vi "Begin.vi"(8 "error in":errorcluster) -> (0 "error out":errorcluster)   [LabVIEW 2017]
doc: "Called before other user functions, this VI is expected to open initial I/O refnums, load in file data, and do all program initialization. Notice that the <B>error out</B> terminal is simply used for data flow. Wiring it to other structures or subVIs ensures that this VI runs first."
uses:
  <vilib>/Rock Robotics/WPI/DriverStation/WPI_DriverStationRobotMode2.ctl
  <vilib>/Rock Robotics/WPI/Joystick/WPI_JoystickDeviceEnum.ctl
  <vilib>/Rock Robotics/WPI/ThirdParty/Phoenix-LabVIEW/Motor Controller/Controls/CTRE_Phoenix_MotorControl_NeutralMode.ctl
  <vilib>/Rock Robotics/WPI/ThirdParty/Phoenix-LabVIEW/Motor Controller/Controls/CTRE_Phoenix_MotorControl_FeedbackDevice.ctl
  Robot Global Data.vi
  <vilib>/Rock Robotics/WPI/ThirdParty/Phoenix-LabVIEW/Pigeon IMU/CTRE_PigeonIMU_Open_TalonSRX.vi
panel:
  in  "Invert? 2":bool=TRUE
  in  "Invert?":bool
  in  "PhaseSensor 2":bool
  in  "PhaseSensor":bool=TRUE
  in  "6 motors?":bool
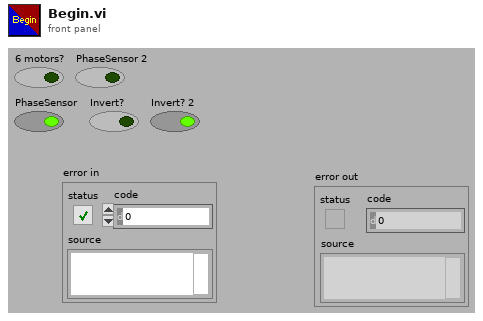
[diagram p1: front panel]
types:
  T1 = typedef "CTRE_Phoenix_MotorControl_FeedbackDevice.ctl" = i8
  T2 = typedef "CTRE_Phoenix_MotorControl_NeutralMode.ctl" = enum8{"EEPROMSetting", "Override to Coast", "Override to Brake"}
  T3 = typedef "WPI_JoystickDeviceEnum.ctl" = enum16{"USB 0", "USB 1", "USB 2", "USB 3", "USB 4", "USB 5"}
  T4 = typedef "WPI_DriverStationRobotMode2.ctl" = enum16{"Autonomous Disabled", "Autonomous Enabled", "Teleop Disabled", "Teleop Enabled", "Disconnected", "Finish", "Test Disabled", "Test Enabled", "Emergency Stopped"}
  T5 = typedef "WPI_MotorControlDeviceRef.ctl" = cluster{"DeviceStatus":errorcluster, "Type":T6, "PWM":cluster{"PWM Channel":T7, "DeadBand":T8}, "CAN":cluster{"Device Number":u8, "SetOutput VI Ref":variant, "GetOutput VI Ref":variant, "Enable VI Ref":variant, "Disable VI Ref":variant, "Data":variant}, "Invert":bool, "DIO PWM":cluster{"PWM \"Enable\" Channel":T7, "DIOChannel":T9, "PWM Rate":dbl}}
  T6 = typedef "WPI_MotorControlType.ctl" = enum16{"PWM", "CAN", "DIO PWM"}
  T7 = typedef "FPGA_DIOPWMChannel.ctl" = enum8{"PWM 0", "PWM 1", "PWM 2", "PWM 3", "PWM 4", "PWM 5", "PWM 6", "PWM 7", "PWM 8", "PWM 9", "PWM MXP 0", "PWM MXP 1", "PWM MXP 2", "PWM MXP 3", "PWM MXP 4", "PWM MXP 5", "PWM MXP 6", "PWM MXP 7", "PWM MXP 8", "PWM MXP 9", "Invalid"}
  T8 = typedef "WPI_PWMDeadband.ctl" = cluster{"Name":string, "maxPositivePwm":i32, "minPositivePwm":i32, "centerPwm":i32, "maxNegativePwm":i32, "minNegativePwm":i32, "angularRange":u16}
  T9 = typedef "FPGA_DIOChannel.ctl" = enum8{"DIO 0", "DIO 1", "DIO 2", "DIO 3", "DIO 4", "DIO 5", "DIO 6", "DIO 7", "DIO 8", "DIO 9", "DIO MXP 0", "DIO MXP 1", "DIO MXP 2", "DIO MXP 3", "DIO MXP 4", "DIO MXP 5", "DIO MXP 6", "DIO MXP 7", "DIO MXP 8", "DIO MXP 9", "DIO MXP 10", "DIO MXP 11", "DIO MXP 12", "DIO MXP 13", "DIO MXP 14", "DIO MXP 15", "SPI Port CS1", "SPI Port CS2", "SPI Port CS3", "SPI Port MISO", "SPI Port MOSI", "Invalid"}
  T10 = typedef "WPI_JoystickDevRef.ctl" = cluster{"Device":T3}
  T11 = typedef "CTRE_PigeonIMU_DeviceRef.ctl" = cluster{"DeviceStatus":errorcluster, "Device Number":u8, "Type":T12, "Device ID":u32, "Handle":u64, "UsageFrame":u32, "Library Path":path}
  T12 = typedef "CTRE_PigeonIMU_ConnectionType.ctl" = u32
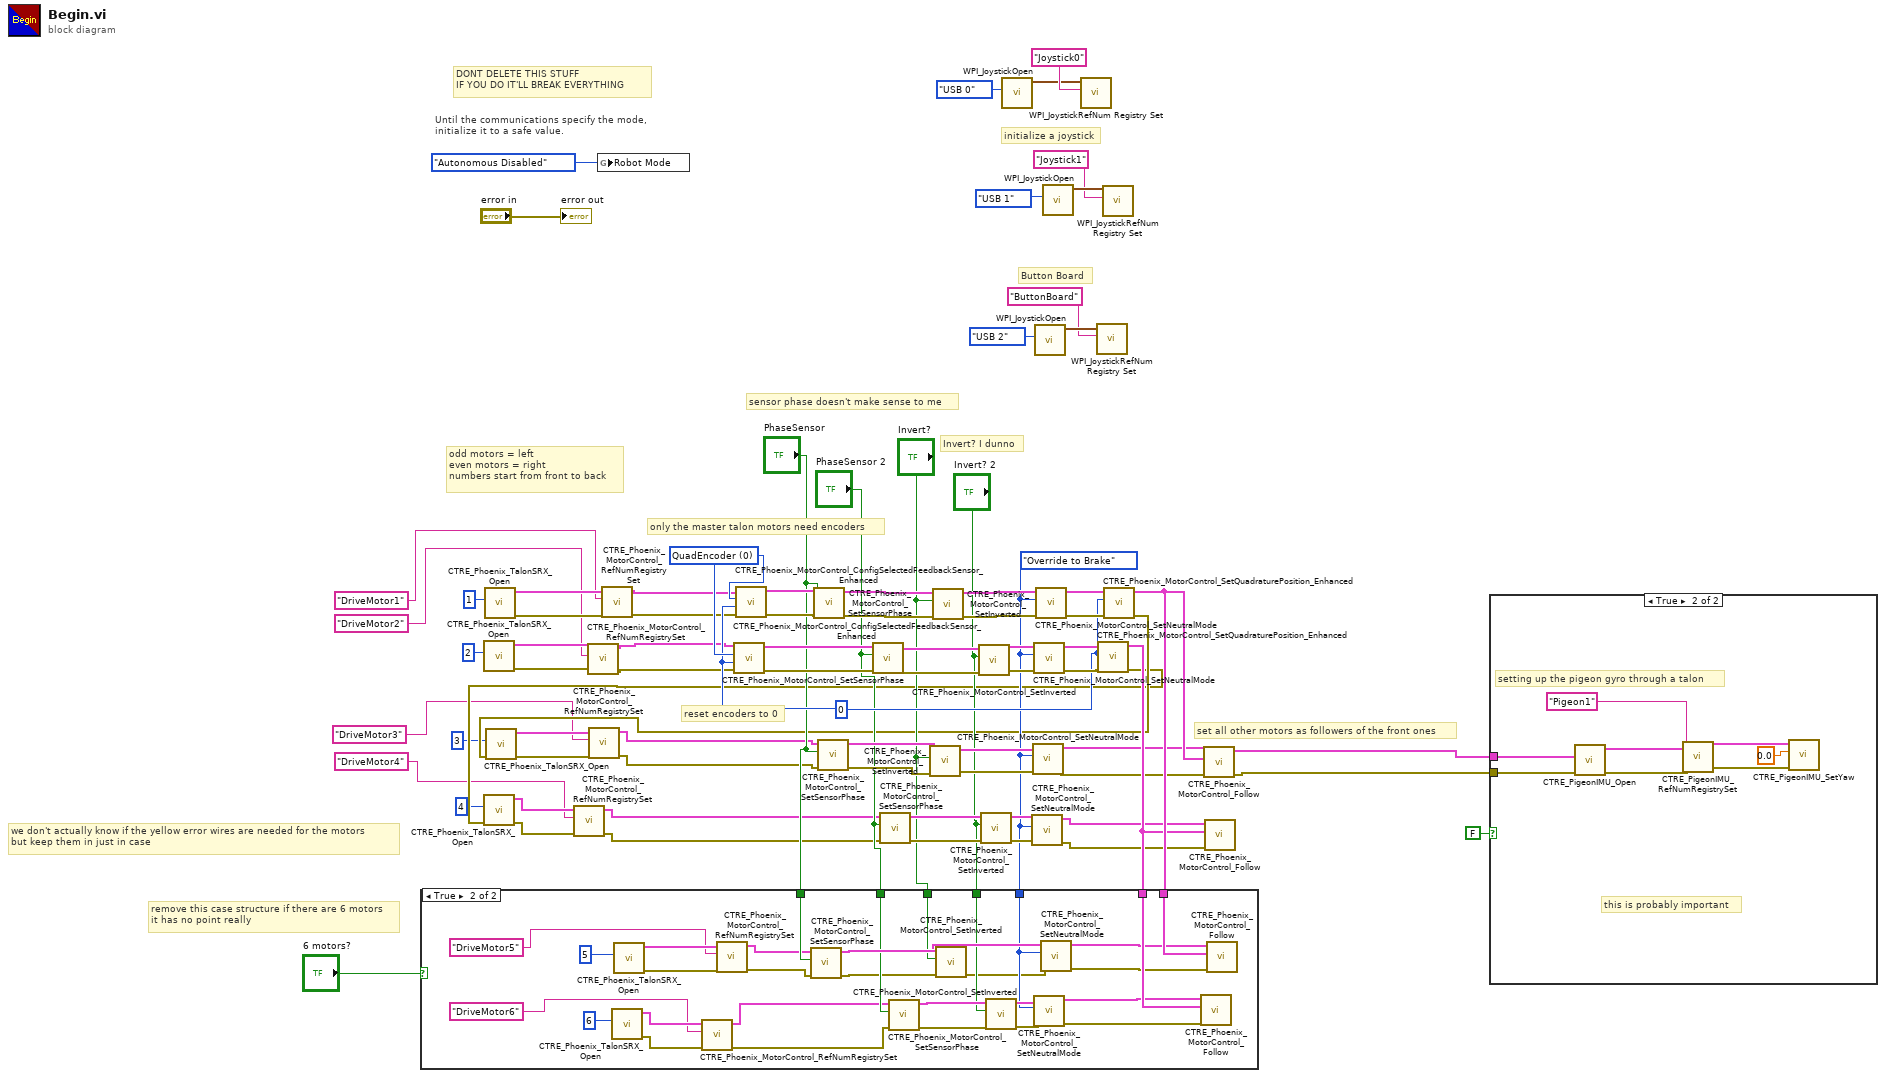
[diagram p0: block diagram]
diagram:
  w48 = 0 ("pidLoopIdx")
  w60 = T1 0 items=["None"=-1, "QuadEncoder"=0, "Analog"=2, "Tachometer"=4, "Pulse Width Encoded Position"=8, "Sensor Sum (S0 + S1)"=9, "Sensor Difference (D0 - D1)"=10, "Remote Source 0"=11, "Remote Source 1"=12, "Software Emulated"=15] ("Feedback Device")
  w36 = CTRE_Phoenix_MotorControl_NeutralMode."Override to Brake" ("Motor Control Neutral Mode")
  # "Invert? I dunno"
  # "sensor phase doesn't make sense to me"
  # "set all other motors as followers of the front ones"
  # "we don't actually know if the yellow error wires are needed for the motors\nbut keep them in just in case"
  # "remove this case structure if there are 6 motors\nit has no point really"
  # "odd motors = left\neven motors = right\nnumbers start from front to back"
  # "reset encoders to 0"
  # "only the master talon motors need encoders"
  # "Button Board"
  # "initialize a joystick"
  # "DONT DELETE THIS STUFF\nIF YOU DO IT'LL BREAK EVERYTHING"
  # "Until the communications specify the mode,\ninitialize it to a safe value."
  n1 = call <vilib>:"CTRE_Phoenix_TalonSRX_Open.vi"("Device Number"=u8 2) -> ("error out"=w10:errorcluster, "CAN Talon SRX Ref"=w21:T5)  [unwired: 9 in]
  n2 = call <vilib>:"CTRE_Phoenix_TalonSRX_Open.vi"("Device Number"=u8 1) -> ("error out"=w9:errorcluster, "CAN Talon SRX Ref"=w22:T5)  [unwired: 9 in]
  n3 = call <vilib>:"CTRE_Phoenix_MotorControl_RefNumRegistrySet.vi"("error in (no error)"=w10, "refnum name"="DriveMotor2", "PhoenixMotorControlDevRef"=w21) -> ("error out"=w17:errorcluster, "PhoenixMotorControlDevRef"=w25:T5)  [unwired: 7 in]
  n4 = global write "Robot Global Data.vi" "Robot Mode"(WPI_DriverStationRobotMode2."Autonomous Disabled" ("Robot Mode")) -> ()
  n5 = call <vilib>:"CTRE_Phoenix_MotorControl_RefNumRegistrySet.vi"("error in (no error)"=w9, "refnum name"="DriveMotor1", "PhoenixMotorControlDevRef"=w22) -> ("error out"=w18:errorcluster, "PhoenixMotorControlDevRef"=w26:T5)  [unwired: 7 in]
  n6 = call <vilib>:"CTRE_Phoenix_MotorControl_ConfigSelectedFeedbackSensor_Enhanced.vi"("error in (no error)"=w17, "pidLoopIdx"=w48, "Feedback Device"=w60, "PhoenixMotorControlDevRef"=w25) -> ("error out"=w54:errorcluster, "PhoenixMotorControlDevRef"=w59:T5)  [unwired: 6 in]
  n7 = call <vilib>:"CTRE_Phoenix_MotorControl_ConfigSelectedFeedbackSensor_Enhanced.vi"("error in (no error)"=w18, "pidLoopIdx"=w48, "Feedback Device"=w60, "PhoenixMotorControlDevRef"=w26) -> ("error out"=w58:errorcluster, "PhoenixMotorControlDevRef"=w47:T5)  [unwired: 6 in]
  n8 = call <vilib>:"CTRE_Phoenix_MotorControl_SetSensorPhase.vi"("error in (no error)"=w58, "PhaseSensor"="PhaseSensor", "PhoenixMotorControlDevRef"=w47) -> ("error out"=w57:errorcluster, "PhoenixMotorControlDevRef"=w46:T5)  [unwired: 7 in]
  n9 = call <vilib>:"CTRE_Phoenix_MotorControl_SetSensorPhase.vi"("error in (no error)"=w54, "PhaseSensor"="PhaseSensor 2", "PhoenixMotorControlDevRef"=w59) -> ("error out"=w53:errorcluster, "PhoenixMotorControlDevRef"=w67:T5)  [unwired: 7 in]
  n10 = call <vilib>:"CTRE_Phoenix_MotorControl_SetInverted.vi"("error in (no error)"=w57, "Invert?"="Invert?", "PhoenixMotorControlDevRef"=w46) -> ("error out"=w56:errorcluster, "PhoenixMotorControlDevRef"=w62:T5)  [unwired: 7 in]
  n11 = call <vilib>:"CTRE_Phoenix_MotorControl_SetInverted.vi"("error in (no error)"=w53, "Invert?"="Invert? 2", "PhoenixMotorControlDevRef"=w67) -> ("error out"=w52:errorcluster, "PhoenixMotorControlDevRef"=w61:T5)  [unwired: 7 in]
  n12 = call <vilib>:"WPI_JoystickOpen.vi"("JoystickDevice"=WPI_JoystickDeviceEnum."USB 0") -> ("JoystickDevRef"=w75:T10)  [unwired: 10 in]
  n13 = call <vilib>:"CTRE_Phoenix_MotorControl_SetNeutralMode.vi"("error in (no error)"=w52, "Motor Control Neutral Mode"=w36, "PhoenixMotorControlDevRef"=w61) -> ("error out"=w51:errorcluster, "PhoenixMotorControlDevRef"=w64:T5)  [unwired: 7 in]
  n14 = call <vilib>:"WPI_JoystickOpen.vi"("JoystickDevice"=WPI_JoystickDeviceEnum."USB 2") -> ("JoystickDevRef"=w73:T10)  [unwired: 10 in]
  n15 = call <vilib>:"CTRE_Phoenix_MotorControl_SetNeutralMode.vi"("error in (no error)"=w56, "Motor Control Neutral Mode"=w36, "PhoenixMotorControlDevRef"=w62) -> ("error out"=w55:errorcluster, "PhoenixMotorControlDevRef"=w66:T5)  [unwired: 7 in]
  n16 = call <vilib>:"WPI_JoystickOpen.vi"("JoystickDevice"=WPI_JoystickDeviceEnum."USB 1") -> ("JoystickDevRef"=w70:T10)  [unwired: 10 in]
  n17 = call <vilib>:"WPI_JoystickRefNum Registry Set.vi"("refnum name"="Joystick0", "JoystickDevRef"=w75) -> ()  [unwired: 8 in, 2 out]
  n18 = call <vilib>:"WPI_JoystickRefNum Registry Set.vi"("refnum name"="ButtonBoard", "JoystickDevRef"=w73) -> ()  [unwired: 8 in, 2 out]
  n19 = call <vilib>:"CTRE_Phoenix_MotorControl_SetQuadraturePosition_Enhanced.vi"("error in (no error)"=w51, "New Position"=w48, "PhoenixMotorControlDevRef"=w64) -> ("error out"=w15:errorcluster, "PhoenixMotorControlDevRef"=w63:T5)  [unwired: 7 in]
  n20 = call <vilib>:"CTRE_Phoenix_TalonSRX_Open.vi"("error in"=w15, "Device Number"=u8 4) -> ("error out"=w11:errorcluster, "CAN Talon SRX Ref"=w19:T5)  [unwired: 8 in]
  n21 = call <vilib>:"CTRE_Phoenix_MotorControl_RefNumRegistrySet.vi"("error in (no error)"=w11, "refnum name"="DriveMotor4", "PhoenixMotorControlDevRef"=w19) -> ("error out"=w12:errorcluster, "PhoenixMotorControlDevRef"=w23:T5)  [unwired: 7 in]
  n22 = call <vilib>:"CTRE_Phoenix_MotorControl_SetSensorPhase.vi"("error in (no error)"=w12, "PhaseSensor"="PhaseSensor 2", "PhoenixMotorControlDevRef"=w23) -> ("error out"=w37:errorcluster, "PhoenixMotorControlDevRef"=w43:T5)  [unwired: 7 in]
  n23 = call <vilib>:"CTRE_Phoenix_MotorControl_SetInverted.vi"("error in (no error)"=w37, "Invert?"="Invert? 2", "PhoenixMotorControlDevRef"=w43) -> ("error out"=w38:errorcluster, "PhoenixMotorControlDevRef"=w39:T5)  [unwired: 7 in]
  n24 = call <vilib>:"CTRE_Phoenix_MotorControl_SetNeutralMode.vi"("error in (no error)"=w38, "Motor Control Neutral Mode"=w36, "PhoenixMotorControlDevRef"=w39) -> ("error out"=w35:errorcluster, "PhoenixMotorControlDevRef"=w34:T5)  [unwired: 7 in]
  n25 = call <vilib>:"WPI_JoystickRefNum Registry Set.vi"("refnum name"="Joystick1", "JoystickDevRef"=w70) -> ()  [unwired: 8 in, 2 out]
  n26 = call <vilib>:"CTRE_Phoenix_MotorControl_SetQuadraturePosition_Enhanced.vi"("error in (no error)"=w55, "New Position"=w48, "PhoenixMotorControlDevRef"=w66) -> ("error out"=w16:errorcluster, "PhoenixMotorControlDevRef"=w65:T5)  [unwired: 7 in]
  n27 = case shown="True" "6 motors?" {
    tunnel: w65 -> [_ w109]
    tunnel: w63 -> [_ w108]
    tunnel: w36 -> [_ w101]
    tunnel: "PhaseSensor" -> [_ w100]
    tunnel: "PhaseSensor 2" -> [_ w99]
    tunnel: "Invert?" -> [_ w98]
    tunnel: "Invert? 2" -> [_ w97]
    frame False {
    }
    frame True {
      n28 = call <vilib>:"CTRE_Phoenix_TalonSRX_Open.vi"("Device Number"=u8 6) -> ("error out"=w87:errorcluster, "CAN Talon SRX Ref"=w89:T5)  [unwired: 9 in]
      n29 = call <vilib>:"CTRE_Phoenix_TalonSRX_Open.vi"("Device Number"=u8 5) -> ("error out"=w88:errorcluster, "CAN Talon SRX Ref"=w90:T5)  [unwired: 9 in]
      n30 = call <vilib>:"CTRE_Phoenix_MotorControl_RefNumRegistrySet.vi"("error in (no error)"=w87, "refnum name"="DriveMotor6", "PhoenixMotorControlDevRef"=w89) -> ("error out"=w79:errorcluster, "PhoenixMotorControlDevRef"=w80:T5)  [unwired: 7 in]
      n31 = call <vilib>:"CTRE_Phoenix_MotorControl_RefNumRegistrySet.vi"("error in (no error)"=w88, "refnum name"="DriveMotor5", "PhoenixMotorControlDevRef"=w90) -> ("error out"=w81:errorcluster, "PhoenixMotorControlDevRef"=w82:T5)  [unwired: 7 in]
      n32 = call <vilib>:"CTRE_Phoenix_MotorControl_SetSensorPhase.vi"("error in (no error)"=w81, "PhaseSensor"=w100, "PhoenixMotorControlDevRef"=w82) -> ("error out"=w96:errorcluster, "PhoenixMotorControlDevRef"=w107:T5)  [unwired: 7 in]
      n33 = call <vilib>:"CTRE_Phoenix_MotorControl_SetSensorPhase.vi"("error in (no error)"=w79, "PhaseSensor"=w99, "PhoenixMotorControlDevRef"=w80) -> ("error out"=w93:errorcluster, "PhoenixMotorControlDevRef"=w106:T5)  [unwired: 7 in]
      n34 = call <vilib>:"CTRE_Phoenix_MotorControl_SetInverted.vi"("error in (no error)"=w96, "Invert?"=w98, "PhoenixMotorControlDevRef"=w107) -> ("error out"=w95:errorcluster, "PhoenixMotorControlDevRef"=w103:T5)  [unwired: 7 in]
      n35 = call <vilib>:"CTRE_Phoenix_MotorControl_SetInverted.vi"("error in (no error)"=w93, "Invert?"=w97, "PhoenixMotorControlDevRef"=w106) -> ("error out"=w92:errorcluster, "PhoenixMotorControlDevRef"=w102:T5)  [unwired: 7 in]
      n36 = call <vilib>:"CTRE_Phoenix_MotorControl_SetNeutralMode.vi"("error in (no error)"=w92, "Motor Control Neutral Mode"=w101, "PhoenixMotorControlDevRef"=w102) -> ("error out"=w91:errorcluster, "PhoenixMotorControlDevRef"=w104:T5)  [unwired: 7 in]
      n37 = call <vilib>:"CTRE_Phoenix_MotorControl_SetNeutralMode.vi"("error in (no error)"=w95, "Motor Control Neutral Mode"=w101, "PhoenixMotorControlDevRef"=w103) -> ("error out"=w94:errorcluster, "PhoenixMotorControlDevRef"=w105:T5)  [unwired: 7 in]
      n38 = call <vilib>:"CTRE_Phoenix_MotorControl_Follow.vi"("error in (no error)"=w91, "Master Controller to Follow"=w108, "PhoenixMotorControlDevRef"=w104) -> ()  [unwired: 7 in, 2 out]
      n39 = call <vilib>:"CTRE_Phoenix_MotorControl_Follow.vi"("error in (no error)"=w94, "Master Controller to Follow"=w109, "PhoenixMotorControlDevRef"=w105) -> ()  [unwired: 7 in, 2 out]
    }
  }
  n40 = call <vilib>:"CTRE_Phoenix_TalonSRX_Open.vi"("error in"=w16, "Device Number"=u8 3) -> ("error out"=w14:errorcluster, "CAN Talon SRX Ref"=w20:T5)  [unwired: 8 in]
  n41 = call <vilib>:"CTRE_Phoenix_MotorControl_RefNumRegistrySet.vi"("error in (no error)"=w14, "refnum name"="DriveMotor3", "PhoenixMotorControlDevRef"=w20) -> ("error out"=w13:errorcluster, "PhoenixMotorControlDevRef"=w24:T5)  [unwired: 7 in]
  n42 = call <vilib>:"CTRE_Phoenix_MotorControl_SetSensorPhase.vi"("error in (no error)"=w13, "PhaseSensor"="PhaseSensor", "PhoenixMotorControlDevRef"=w24) -> ("error out"=w42:errorcluster, "PhoenixMotorControlDevRef"=w44:T5)  [unwired: 7 in]
  n43 = call <vilib>:"CTRE_Phoenix_MotorControl_SetInverted.vi"("error in (no error)"=w42, "Invert?"="Invert?", "PhoenixMotorControlDevRef"=w44) -> ("error out"=w40:errorcluster, "PhoenixMotorControlDevRef"=w41:T5)  [unwired: 7 in]
  n44 = call <vilib>:"CTRE_Phoenix_MotorControl_SetNeutralMode.vi"("error in (no error)"=w40, "Motor Control Neutral Mode"=w36, "PhoenixMotorControlDevRef"=w41) -> ("error out"=w32:errorcluster, "PhoenixMotorControlDevRef"=w33:T5)  [unwired: 7 in]
  n45 = call <vilib>:"CTRE_Phoenix_MotorControl_Follow.vi"("error in (no error)"=w32, "Master Controller to Follow"=w65, "PhoenixMotorControlDevRef"=w33) -> ("error out"=w49:errorcluster, "PhoenixMotorControlDevRef"=w50:T5)  [unwired: 7 in]
  n46 = call <vilib>:"CTRE_Phoenix_MotorControl_Follow.vi"("error in (no error)"=w35, "Master Controller to Follow"=w63, "PhoenixMotorControlDevRef"=w34) -> ()  [unwired: 7 in, 2 out]
  n47 = case shown="True" FALSE {
    tunnel: w50 -> [_ w111]
    tunnel: w49 -> [_ w110]
    frame False {
    }
    frame True {
      # "this is probably important"
      # "setting up the pigeon gyro through a talon"
      n48 = call-poly <vilib>:"CTRE_PigeonIMU_Open.vi"("error in"=w110, "CAN Talon SRX Ref"=w111) -> ("error out"=w116:errorcluster, "PigeonIMUDevRef"=w117:T11)  [unwired: 8 in]
      n49 = call <vilib>:"CTRE_PigeonIMU_RefNumRegistrySet.vi"("error in (no error)"=w116, "refnum name"="Pigeon1", "PigeonIMUDevRef"=w117) -> ("error out"=w113:errorcluster, "PigeonIMUDevRef"=w114:T11)  [unwired: 7 in]
      n50 = call <vilib>:"CTRE_PigeonIMU_SetYaw.vi"("error in (no error)"=w113, "Value"=0.0, "PigeonIMUDevRef"=w114) -> ()  [unwired: 7 in, 2 out]
    }
  }
  "error out" <- "error in"
